vi "Actor Core.vi"(8 "error in":errorcluster, 11 "H3611i Actor in":refnum<class "H3611i Actor.lvclass">) -> (0 "error out":errorcluster, 3 "Actor out":refnum<class "Actor.lvclass">)   [LabVIEW 2018, in "H3611i.lvlib" / "H3611i Actor.lvclass"]
doc: "(<B>Filename</B>: Actor Framework.lvlib:Actor.lvclass:Actor Core.vi)\n\nReceives messages to the actor, reacts to them, and initiates any error handling that may shut the actor down.\n\nDescendant classes may override this VI to append parallel tasks for the actor to complete while it handles messages. Overrides use the Call Parent Method node."
uses:
  H3611i Actor.lvclass
  C:/Program Files (x86)/National Instruments/LabVIEW 2018/vi.lib/ActorFramework/Actor/Actor.lvclass
  <vilib>/ActorFramework/Actor/Actor.lvclass
  <vilib>/ActorFramework/Actor/Actor.lvclass/Actor.ctl
  <vilib>/ActorFramework/Message Enqueuer/Message Enqueuer.lvclass/Message Enqueuer.ctl
  H3611i Actor.lvclass/H3611i Actor.ctl
  <vilib>/ActorFramework/Stop Msg/Stop Msg.lvclass/Stop Msg.ctl
  <vilib>/ActorFramework/Message Enqueuer/Init from Existing Queue.vi
  <vilib>/ActorFramework/Message Enqueuer/Enqueue.vi
  <vilib>/ActorFramework/Message Enqueuer/Enqueue Critical.vi
  H3611i Actor Messages/Measure H3611i Range Msg/Measure H3611i Range Msg.lvclass
  C:/Program Files (x86)/National Instruments/LabVIEW 2018/vi.lib/ActorFramework/Message/Message.lvclass
  <vilib>/ActorFramework/Stop Msg/Stop Msg.lvclass
  <vilib>/ActorFramework/Message Priority Queue/Priority Enqueue.vi
  Sensor Actor/Sensor/Sensor.lvclass
  <vilib>/ActorFramework/Message Enqueuer/Message Enqueuer.lvclass
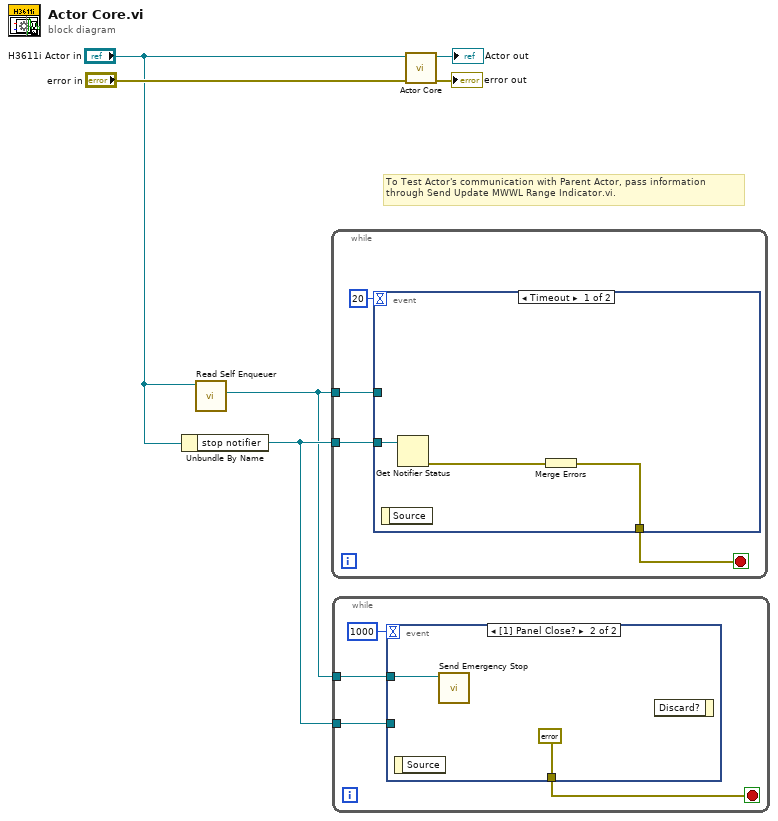
[diagram p0: block diagram]
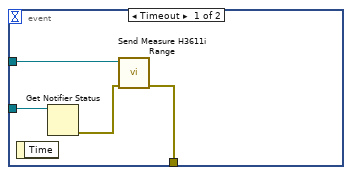
[diagram p2: hidden frame]
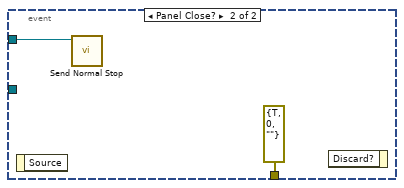
[diagram p3: hidden frame]
diagram:
  # "To Test Actor's communication with Parent Actor, pass information\nthrough Send Update MWWL Range Indicator.vi."
  n1 = Unbundle By Name("H3611i Actor in") -> ("stop notifier"=w2:refnum<notifier>)
  n2 = call <vilib>:"Read Self Enqueuer.vi"("Actor"="H3611i Actor in") -> ("Self Enqueuer"=w1:refnum<class "Message Enqueuer.lvclass">)  [unwired: 10 in]
  n3 = while {
    tunnel: w2 -> [w9]
    tunnel: w1 -> [w8]
    stop <- w7 stop-if-true
    n4 = event shown="[0] Timeout" {
      selector: _ -> [_ _]
      dyn-events: _ -> [_ _]
      timeout: 20 -> [_ _]
      tunnel: w9 -> [w13 _]
      tunnel: w8 -> [_ w15]
      tunnel: [w11 errorcluster {"status"=TRUE, "code"=0, "source"=""} ("error IO")] -> w7
      event Timeout {
        n5 = event-data() -> ()  [unwired: 1 in, 1 out]
        n6 = Get Notifier Status(notifier=w13) -> (error out=w12:errorcluster)  [unwired: 1 in, 4 out]
        n7 = Merge Errors(w12) -> (w11:errorcluster)
      }
      event Panel Close? {
        n8 = event-data() -> ()  [unwired: 1 in, 1 out]
        n9 = call <vilib>:"Send Normal Stop.vi"("Message Enqueuer"=w15) -> ()  [unwired: 10 in, 1 out]
        n10 = event-data() -> ()  [unwired: 2 in, 1 out]
      }
    }
  }
  n11 = while {
    tunnel: w2 -> [w17]
    tunnel: w1 -> [w16]
    stop <- w18 stop-if-true
    n12 = event shown="[1] Panel Close?" {
      selector: _ -> [_ _]
      dyn-events: _ -> [_ _]
      timeout: 1000 -> [_ _]
      tunnel: [w20 errorcluster {"status"=TRUE, "code"=0, "source"=""} ("error out")] -> w18
      tunnel: w17 -> [w23 _]
      tunnel: w16 -> [w22 w25]
      event Timeout {
        n13 = event-data() -> ()  [unwired: 1 in, 1 out]
        n14 = Get Notifier Status(notifier=w23) -> (error out=w21:errorcluster)  [unwired: 1 in, 4 out]
        n15 = call "Send Measure H3611i Range.vi"("error in (no error)"=w21, "Message Enqueuer in"=w22) -> ("error out"=w20:errorcluster)  [unwired: 8 in, 1 out]
      }
      event Panel Close? {
        n16 = event-data() -> ()  [unwired: 1 in, 1 out]
        n17 = call <vilib>:"Send Emergency Stop.vi"("Message Enqueuer"=w25) -> ()  [unwired: 10 in, 1 out]
        n18 = event-data() -> ()  [unwired: 2 in, 1 out]
      }
    }
  }
  n19 = call-parent "Actor Core.vi"("error in"="error in", "Sensor in"="H3611i Actor in") -> ("error out"=→"error out":errorcluster, "Actor out"=→"Actor out":refnum<class "Actor.lvclass">)  [unwired: 8 in]
